vi "get camera driver.vi"(8 "error in (no error)":errorcluster, 9 "Path":path, 10 "Section":string, 11 "abstract camera driver factory in":refnum<class "abstract camera driver factory.lvclass">) -> (0 "error out":errorcluster, 2 "Camera Driver.lvclass":refnum<class "Camera Driver.lvclass">)   [LabVIEW 2022 SP3, in "abstract camera driver factory.lvclass"]
uses:
  abstract camera driver factory.lvclass
  Camera Driver/Camera Driver.lvclass
  abstract camera driver factory.lvclass/abstract camera driver factory.ctl
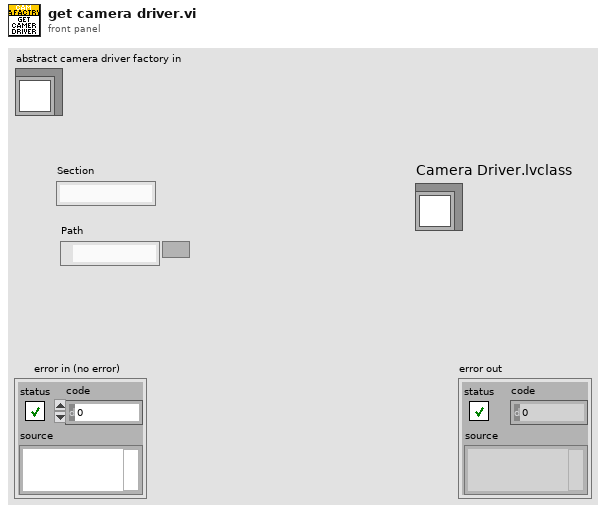
[diagram p1: front panel]
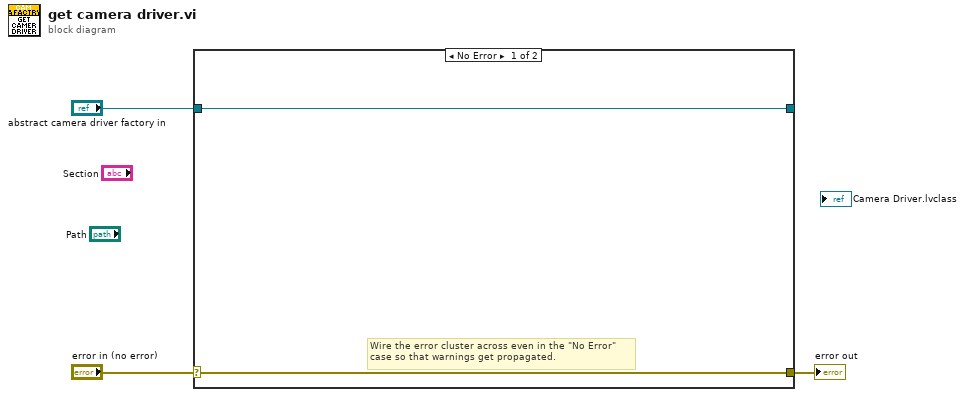
[diagram p0: block diagram]
diagram:
  n1 = case shown="No Error" "error in (no error)" {
    selector: "error in (no error)" -> [w4 w7]
    tunnel: [w4 w7] -> w2
    tunnel: [w5 w6] -> _
    tunnel: "abstract camera driver factory in" -> [w5 w6]
    frame No Error {
      # "Wire the error cluster across even in the \"No Error\"\ncase so that warnings get propagated."
    }
    frame Error {
    }
  }
  "error out" <- w2
